vi "标样核查.vi"(11 "标样核查配置":T1={"数据保存间隔"=1.0, "水温标样值"=0.0, "pH标样值"=0.0, "溶解氧标样值"=0.0, "电导率标样值"=0.0, "浊度标样值"=0.0}) -> ()   [LabVIEW 2016, in "斯坦道多参数.lvlib"]
panel:
  out "运行状态":u16(ring) items=["空闲", "水样测试", "标样核查"]
  out "seconds since 1Jan1904":timestamp
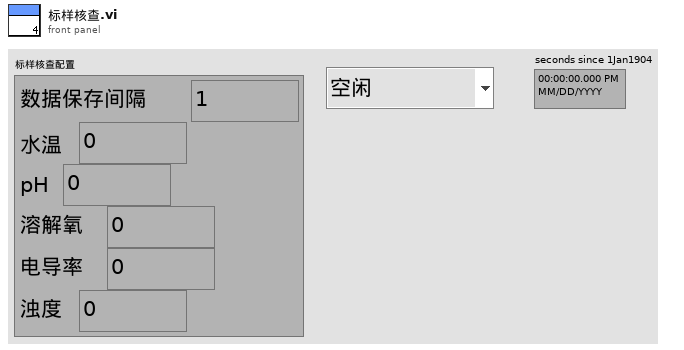
[diagram p1: front panel]
types:
  T1 = cluster{"数据保存间隔":dbl, "水温标样值":dbl, "pH标样值":dbl, "溶解氧标样值":dbl, "电导率标样值":dbl, "浊度标样值":dbl}
  T2 = cluster{"因子编码":string, "单位":string, "标样参考值":sgl, "水样数据时间":timestamp, "水样实测值":sgl, "水样数据标识":string, "探头温度":sgl}
  T3 = typedef "LVDateTimeRec.ctl" = cluster{"秒数的小数部分":dbl, "秒":i32, "分":i32, "时":i32, "日":i32, "月":i32, "年":i32, "天数（周）":i32, "天数（年）":i32, "DST":i32}
  T4 = cluster{"CH":u16, "监测值":dbl, "监测信号值":dbl, "温度偏移修正值":sgl}
  T5 = cluster{"电极状态标志":u16, "电极型号标志":u16, "酸碱度测量值":sgl, "温度测量值":sgl, "酸碱度信号值":sgl, "温度信号值":sgl, "酸碱度偏移修正值":sgl, "温度偏移修正值":sgl, "手动温度补偿值":sgl, "酸碱度电极零点":sgl, "酸碱度电极斜率":sgl, "第1点标准值记录":sgl, "第1点信号值记录":sgl, "第1点温度值记录":sgl, "第2点标准值记录":sgl, "第2点信号值记录":sgl, "第2点温度值记录":sgl, "命令滤波设定":u16, "温度模式":enum16{"ATC", "MTC"}, "生产批次":u16, "电极序号":u16, "串口地址":u16, "串口波特率":enum16{"9600", "19200", "115200"}, "串口校验位":enum16{"NONE", "ODD", "EVEN"}, "串口停止位":enum16{"1bit", "2bit"}, "第一点标准值":sgl, "第二点标准值":sgl}
  T6 = cluster{"电极状态标志":u16, "电极型号标志":u16, "溶解氧测量值":sgl, "温度测量值":sgl, "溶解氧饱和度值":sgl, "盐度补偿值":sgl, "大气压补偿值":sgl, "溶解氧偏移修正值":sgl, "温度偏移修正值":sgl, "手动温度补偿值":sgl, "溶解氧电极零点":sgl, "溶解氧电极斜率":sgl, "第1点标准值记录":sgl, "第1点信号值记录":sgl, "第1点温度值记录":sgl, "第2点标准值记录":sgl, "第2点信号值记录":sgl, "第2点温度值记录":sgl, "命令滤波设定":u16, "温度模式":enum16{"ATC", "MTC"}, "生产批次":u16, "电极序号":u16, "串口地址":u16, "串口波特率":enum16{"9600", "19200", "115200"}, "串口校验位":enum16{"NONE", "ODD", "EVEN"}, "串口停止位":enum16{"1bit", "2bit"}, "第一点标准值":sgl, "第二点标准值":sgl}
  T7 = cluster{"电极状态标志":u16, "电极型号标志":u16, "电导率测量值":sgl, "温度测量值":sgl, "电导率信号值":sgl, "温度信号值":sgl, "温度补偿系数":sgl, "电导率偏移修正值":sgl, "温度偏移修正值":sgl, "手动温度补偿值":sgl, "电导率电极零点":sgl, "电导率电极斜率":sgl, "命令滤波设定":u16, "温度模式":enum16{"ATC", "MTC"}, "生产批次":u16, "电极序号":u16, "串口地址":u16, "串口波特率":enum16{"9600", "19200", "115200"}, "串口校验位":enum16{"NONE", "ODD", "EVEN"}, "串口停止位":enum16{"1bit", "2bit"}, "第一点标准值":sgl, "第二点标准值":sgl}
  T8 = cluster{"电极状态标志":u16, "电极型号标志":u16, "浊度测量值":sgl, "温度测量值":sgl, "浊度信号值":sgl, "浊度偏移修正值":sgl, "温度偏移修正值":sgl, "手动温度补偿值":sgl, "浊度电极零点":sgl, "浊度电极斜率":sgl, "第1点标准值记录":sgl, "第1点信号值记录":sgl, "第1点温度值记录":sgl, "第2点标准值记录":sgl, "第2点信号值记录":sgl, "第2点温度值记录":sgl, "命令滤波设定":u16, "温度模式":enum16{"ATC", "MTC"}, "生产批次":u16, "电极序号":u16, "串口地址":u16, "串口波特率":enum16{"9600", "19200", "115200"}, "串口校验位":enum16{"NONE", "ODD", "EVEN"}, "串口停止位":enum16{"1bit", "2bit"}, "第一点标准值":sgl, "第二点标准值":sgl}
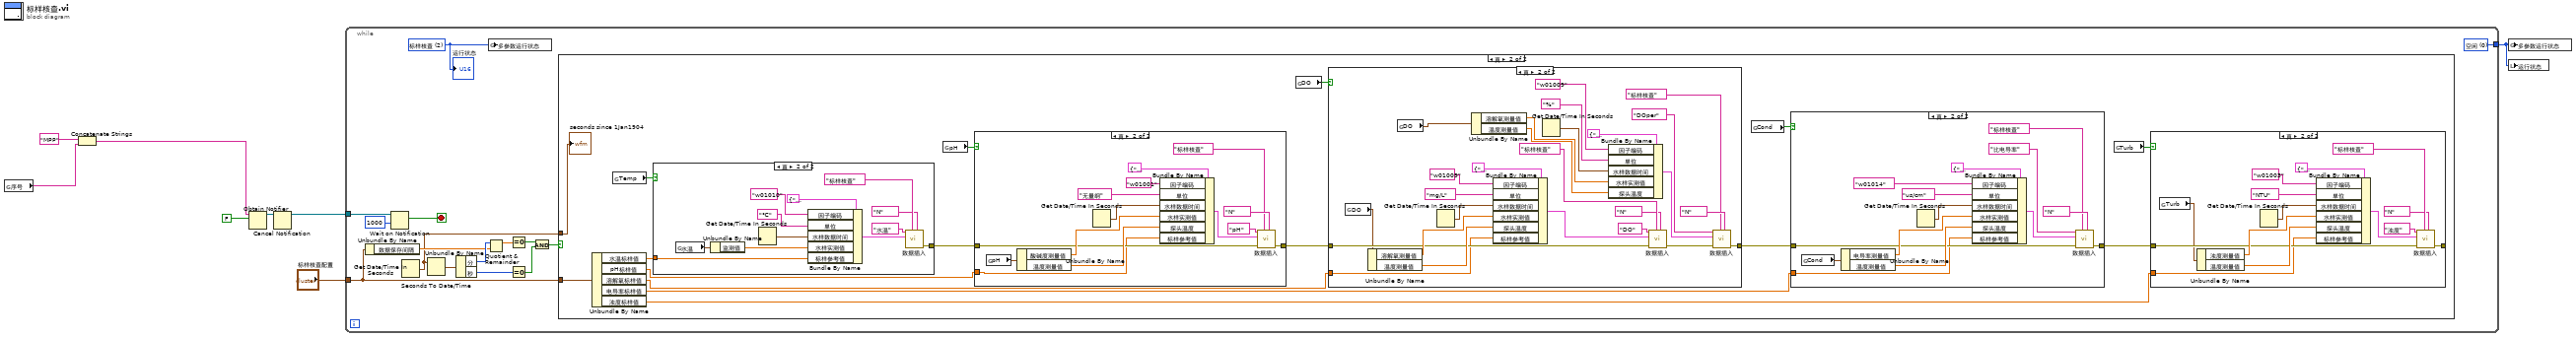
[diagram p0: block diagram]
diagram:
  n1 = global read "多参数全局变量.vi" "序号"() -> (w1:string)
  n2 = Concatenate Strings("MPP" ("名称（未命名）"), w1) -> (w2:string)
  n3 = Obtain Notifier(name (unnamed)=w2, notification data type=FALSE) -> (notifier out=w5:refnum<notifier>)  [unwired: 2 in, 2 out]
  n4 = Cancel Notification(0:w5) -> (8:w4:refnum<notifier>)  [unwired: 1 in, 2 out]
  n5 = while {
    tunnel: "标样核查配置" -> [w19]
    tunnel: [w13] -> w3
    tunnel: w4 -> [w12]
    stop <- w10 stop-if-true
    w13 = u16 0 items=["空闲", "水样测试", "标样核查"] ("多参数运行状态")
    w9 = u16 2 items=["空闲", "水样测试", "标样核查"] ("多参数运行状态")
    n6 = Unbundle By Name(w19) -> ("数据保存间隔"=w17:dbl)
    n7 = Wait on Notification(notifier=w12, timeout in ms (-1)=1000 ("超时毫秒(-1)")) -> (notification=w10:bool)  [unwired: 2 in, 3 out]
    n8 = Get Date/Time In Seconds() -> (seconds since 1Jan1904=w14:timestamp)
    n9 = Seconds To Date/Time(time stamp (now)=w14) -> (date time rec=w23:T3)  [unwired: 1 in]
    n10 = Unbundle By Name(w23) -> ("分"=w18:i32, "秒"=w22:i32)
    n11 = Quotient & Remainder(x=w18, y=w17) -> (x-y*floor(x/y)=w16:dbl)  [unwired: 1 out]
    n12 = global write "多参数全局变量.vi" "多参数运行状态"(w9) -> ()
    n13 = Equal To 0?(x=w16) -> (x = 0?=w15:bool)
    n14 = Equal To 0?(x=w22) -> (x = 0?=w21:bool)
    n15 = And(x=w15, y=w21) -> (x .and. y?=w20:bool)
    n16 = case shown="真" w20 {
      tunnel: w19 -> [_ w29]
      tunnel: w14 -> [_ w39]
      frame False {
      }
      frame True {
        n17 = Unbundle By Name(w29) -> ("水温标样值"=w28:dbl, "pH标样值"=w27:dbl, "溶解氧标样值"=w26:dbl, "电导率标样值"=w25:dbl, "浊度标样值"=w24:dbl)
        n18 = global read "断电保存变量.vi" "Temp"() -> (w34:bool)
        n19 = case shown="真" w34 {
          tunnel: [_ w109] -> w38
          tunnel: w28 -> [_ w108]
          frame False {
          }
          frame True {
            n20 = global read "国弘过程全局变量.vi" "水温"() -> (w118:T4)
            n21 = Unbundle By Name(w118) -> ("监测值"=w117:dbl)
            n22 = Get Date/Time In Seconds() -> (seconds since 1Jan1904=w116:timestamp)
            n23 = Bundle By Name(cluster=T2 {"因子编码"="w01003", "单位"="无量纲", "标样参考值"=0.0, "水样数据时间"=timestamp(0 s since 1904-01-01), "水样实测值"=0.0, "水样数据标识"="N", "探头温度"=0.0} ("data in"), "因子编码"="w01010", "单位"="℃", "水样数据时间"=w116, "水样实测值"=w117, "标样参考值"=w108) -> (w115:T2)
            n24 = call "数据插入.vi"("数据标记表"="N", "测量模式"="标样核查", "data in"=w115, "table输入"="水温") -> ("error out"=w109:errorcluster)  [unwired: 7 in]
          }
        }
        n25 = global read "断电保存变量.vi" "pH"() -> (w33:bool)
        n26 = case shown="真" w33 {
          tunnel: w38 -> [_ w96]
          tunnel: [_ w95] -> w37
          tunnel: w27 -> [_ w94]
          frame False {
          }
          frame True {
            n27 = global read "国弘过程全局变量.vi" "pH"() -> (w102:T5)
            n28 = Unbundle By Name(w102) -> ("酸碱度测量值"=w103:sgl, "温度测量值"=w100:sgl)
            n29 = Get Date/Time In Seconds() -> (seconds since 1Jan1904=w104:timestamp)
            n30 = Bundle By Name(cluster=T2 {"因子编码"="w01003", "单位"="无量纲", "标样参考值"=0.0, "水样数据时间"=timestamp(0 s since 1904-01-01), "水样实测值"=0.0, "水样数据标识"="N", "探头温度"=0.0} ("data in"), "因子编码"="w01001", "单位"="无量纲", "水样数据时间"=w104, "水样实测值"=w103, "探头温度"=w100, "标样参考值"=w94) -> (w105:T2)
            n31 = call "数据插入.vi"("数据标记表"="N", "测量模式"="标样核查", "error in (no error)"=w96, "data in"=w105, "table输入"="pH") -> ("error out"=w95:errorcluster)  [unwired: 6 in]
          }
        }
        n32 = global read "断电保存变量.vi" "DO"() -> (w32:bool)
        n33 = case shown="真" w32 {
          tunnel: w37 -> [_ w83]
          tunnel: [_ w80] -> w36
          tunnel: w26 -> [_ w82]
          frame False {
          }
          frame True {
            n34 = global read "国弘过程全局变量.vi" "DO"() -> (w68:T6)
            n35 = Unbundle By Name(w68) -> ("溶解氧测量值"=w91:sgl, "温度测量值"=w93:sgl)
            n36 = global read "国弘过程全局变量.vi" "DO"() -> (w69:T6)
            n37 = Get Date/Time In Seconds() -> (seconds since 1Jan1904=w90:timestamp)
            n38 = Unbundle By Name(w69) -> ("溶解氧测量值"=w73:sgl, "温度测量值"=w71:sgl)
            n39 = Bundle By Name(cluster=T2 {"因子编码"="w01003", "单位"="无量纲", "标样参考值"=0.0, "水样数据时间"=timestamp(0 s since 1904-01-01), "水样实测值"=0.0, "水样数据标识"="N", "探头温度"=0.0} ("data in"), "因子编码"="w01009", "单位"="mg/L", "水样数据时间"=w90, "水样实测值"=w91, "探头温度"=w93, "标样参考值"=w82) -> (w89:T2)
            n40 = Get Date/Time In Seconds() -> (seconds since 1Jan1904=w74:timestamp)
            n41 = Bundle By Name(cluster=T2 {"因子编码"="w01003", "单位"="无量纲", "标样参考值"=0.0, "水样数据时间"=timestamp(0 s since 1904-01-01), "水样实测值"=0.0, "水样数据标识"="N", "探头温度"=0.0} ("data in"), "因子编码"="w01009", "单位"="%", "水样数据时间"=w74, "水样实测值"=w73, "探头温度"=w71) -> (w70:T2)
            n42 = call "数据插入.vi"("数据标记表"="N", "测量模式"="标样核查", "error in (no error)"=w83, "data in"=w89, "table输入"="DO") -> ("error out"=w81:errorcluster)  [unwired: 6 in]
            n43 = call "数据插入.vi"("数据标记表"="N", "测量模式"="标样核查", "error in (no error)"=w81, "data in"=w70, "table输入"="DOper") -> ("error out"=w80:errorcluster)  [unwired: 6 in]
          }
        }
        n44 = global read "断电保存变量.vi" "Cond"() -> (w31:bool)
        n45 = case shown="真" w31 {
          tunnel: w36 -> [_ w56]
          tunnel: [_ w55] -> w35
          tunnel: w25 -> [_ w54]
          frame False {
          }
          frame True {
            n46 = global read "国弘过程全局变量.vi" "Cond"() -> (w62:T7)
            n47 = Unbundle By Name(w62) -> ("电导率测量值"=w63:sgl, "温度测量值"=w60:sgl)
            n48 = Get Date/Time In Seconds() -> (seconds since 1Jan1904=w64:timestamp)
            n49 = Bundle By Name(cluster=T2 {"因子编码"="w01003", "单位"="无量纲", "标样参考值"=0.0, "水样数据时间"=timestamp(0 s since 1904-01-01), "水样实测值"=0.0, "水样数据标识"="N", "探头温度"=0.0} ("data in"), "因子编码"="w01014", "单位"="us/cm", "水样数据时间"=w64, "水样实测值"=w63, "探头温度"=w60, "标样参考值"=w54) -> (w65:T2)
            n50 = call "数据插入.vi"("数据标记表"="N", "测量模式"="标样核查", "error in (no error)"=w56, "data in"=w65, "table输入"="比电导率") -> ("error out"=w55:errorcluster)  [unwired: 6 in]
          }
        }
        n51 = global read "断电保存变量.vi" "Turb"() -> (w30:bool)
        n52 = case shown="真" w30 {
          tunnel: w35 -> [_ w43]
          tunnel: [_ w42] -> _
          tunnel: w24 -> [_ w41]
          frame False {
          }
          frame True {
            n53 = global read "国弘过程全局变量.vi" "Turb"() -> (w40:T8)
            n54 = Unbundle By Name(w40) -> ("浊度测量值"=w51:sgl, "温度测量值"=w53:sgl)
            n55 = Get Date/Time In Seconds() -> (seconds since 1Jan1904=w50:timestamp)
            n56 = Bundle By Name(cluster=T2 {"因子编码"="w01003", "单位"="无量纲", "标样参考值"=0.0, "水样数据时间"=timestamp(0 s since 1904-01-01), "水样实测值"=0.0, "水样数据标识"="N", "探头温度"=0.0} ("data in"), "因子编码"="w01003", "单位"="NTU", "水样数据时间"=w50, "水样实测值"=w51, "探头温度"=w53, "标样参考值"=w41) -> (w49:T2)
            n57 = call "数据插入.vi"("数据标记表"="N", "测量模式"="标样核查", "error in (no error)"=w43, "data in"=w49, "table输入"="浊度") -> ("error out"=w42:errorcluster)  [unwired: 6 in]
          }
        }
        "seconds since 1Jan1904" <- w39
      }
    }
    "运行状态" <- w9
  }
  n58 = global write "多参数全局变量.vi" "多参数运行状态"(w3) -> ()
  n59 = local write "运行状态"(w3) -> ()
